vi "fk.vi"(8 "error in (no error)":errorcluster, 10 "Theta 1":dbl, 11 "Theta 0":dbl) -> (0 "error out":errorcluster, 2 "Link2Y":dbl, 3 "Link2X":dbl, 5 "Link1Y":dbl, 7 "Link1X":dbl)   [LabVIEW 2017]
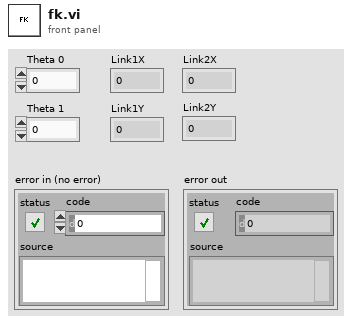
[diagram p1: front panel]
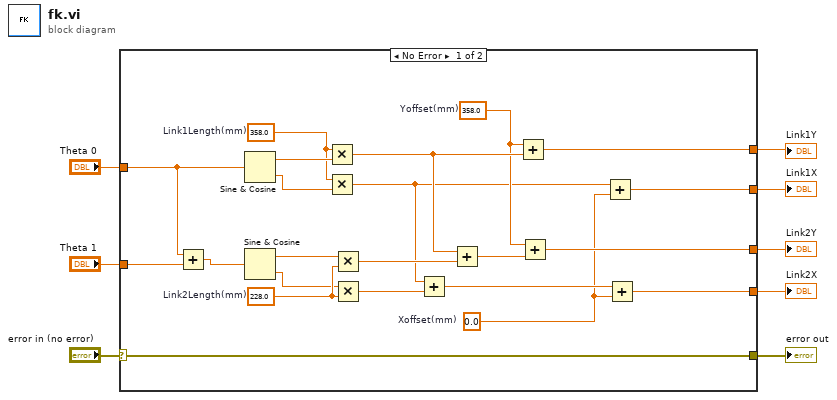
[diagram p0: block diagram]
diagram:
  n1 = case shown="No Error" "error in (no error)" {
    selector: "error in (no error)" -> [w9 w31]
    tunnel: [w9 w31] -> w7
    tunnel: "Theta 0" -> [w22 _]
    tunnel: "Theta 1" -> [w21 _]
    tunnel: [w16 _] -> w4
    tunnel: [w15 _] -> w3
    tunnel: [w11 _] -> w2
    tunnel: [w10 _] -> w1
    frame No Error {
      w12 = 0.0  # Xoffset(mm)
      w17 = 358.0  # Yoffset(mm)
      w26 = 228.0  # Link2Length(mm)
      w29 = 358.0  # Link1Length(mm)
      n2 = Add(x=w22, y=w21) -> (x+y=w20:dbl)
      n3 = Sine & Cosine(0:w22) -> (1:w30:dbl, 2:w28:dbl)
      n4 = Sine & Cosine(0:w20) -> (1:w27:dbl, 2:w25:dbl)
      n5 = Multiply(x=w29, y=w30) -> (x*y=w19:dbl)
      n6 = Multiply(x=w29, y=w28) -> (x*y=w14:dbl)
      n7 = Multiply(x=w27, y=w26) -> (x*y=w23:dbl)
      n8 = Multiply(x=w25, y=w26) -> (x*y=w24:dbl)
      n9 = Add(x=w14, y=w24) -> (x+y=w13:dbl)
      n10 = Add(x=w19, y=w23) -> (x+y=w18:dbl)
      n11 = Add(x=w17, y=w19) -> (x+y=w16:dbl)
      n12 = Add(x=w17, y=w18) -> (x+y=w15:dbl)
      n13 = Add(x=w14, y=w12) -> (x+y=w11:dbl)
      n14 = Add(x=w13, y=w12) -> (x+y=w10:dbl)
    }
    frame Error {
    }
  }
  "error out" <- w7
  "Link1Y" <- w4
  "Link2Y" <- w3
  "Link1X" <- w2
  "Link2X" <- w1
